vi "Digital_Counter_w_External_Clock_V2.vi"() -> ()   [LabVIEW 2020]
uses:
  <vilib>/Utility/error.llb/DialogType.ctl
  <vilib>/DAQmx/create/channels.llb/DAQmx Create Channel (CO-Pulse Generation-Frequency).vi
  <vilib>/DAQmx/configure/timing.llb/DAQmx Timing (Implicit).vi
panel:
  out "Feet Traveled":u64
  in  "stop":bool
  out "Pulse Count":u64
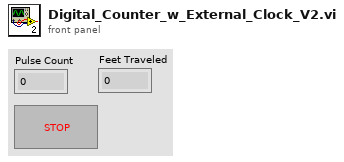
[diagram p1: front panel]
types:
  T1 = typedef "DialogType.ctl" = u16
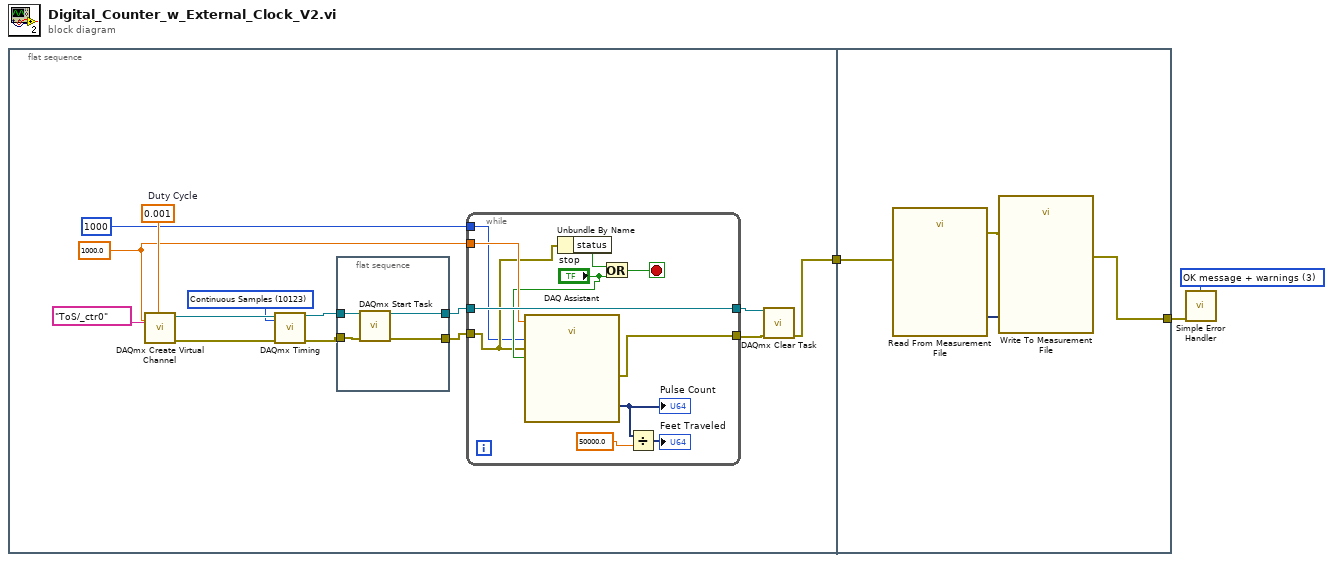
[diagram p0: block diagram]
diagram:
  w3 = T1 3 items=["no dialog", "OK message", "continue or stop message", "OK message + warnings", "continue/stop + warnings"] ("type of dialog (OK msg:1)")
  n1 = flat-sequence {
    tunnel: [w4] -> w2
    tunnel: w2 -> [w34]
    tunnel: [w33] -> w1
    frame #0 {
      w7 = 1000.0 ("Rate (Hz)")
      w13 = 0.001  # Duty Cycle
      w15 = 10123 items=["Finite Samples"=10178, "Continuous Samples"=10123] ("sample mode")
      n2 = call-poly <vilib>:"DAQmx Create Virtual Channel.vi"("frequency"=w7, "duty cycle"=w13, "counter"=tag "ToS/_ctr0" ("Sample Clock Src")) -> ("task out"=w16:refnum<k21>, "error out"=w17:errorcluster)  [unwired: 11 in]
      n3 = call-poly <vilib>:"DAQmx Timing.vi"("task/channels in"=w16, "sample mode"=w15, "error in"=w17) -> ("task out"=w12:refnum<k21>, "error out"=w11:errorcluster)  [unwired: 11 in]
      n4 = flat-sequence {
        tunnel: w12 -> [w32]
        tunnel: w11 -> [w31]
        tunnel: [w30] -> w10
        tunnel: [w29] -> w9
        frame #0 {
          n5 = call <vilib>:"DAQmx Start Task.vi"("task/channels in"=w32, "error in"=w31) -> ("task out"=w30:refnum<k21>, "error out"=w29:errorcluster)  [unwired: 12 in]
        }
      }
      n6 = while {
        tunnel: w10 -> [w28]
        tunnel: w9 -> [w24]
        tunnel: [w28] -> w8
        tunnel: w7 -> [w27]
        tunnel: 1000 ("number of samples") -> [w23]
        tunnel: [w21] -> w5
        stop <- w22 stop-if-true
        n7 = call "DAQ Assistant"("rate"=w27, "number of samples"=w23, "error in"=w24, "stop (F)"="stop") -> ("data"=w19:dynamicdata, "error out"=w21:errorcluster)  [unwired: 12 in, 2 out]
        "Pulse Count" <- w19
        n8 = Unbundle By Name(w24) -> ("status"=w26:bool)
        n9 = Or(x=w26, y="stop") -> (x .or. y?=w22:bool)
        n10 = Divide(x=w19, y=50000.0) -> (x/y=→"Feet Traveled":dynamicdata)
      }
      n11 = call <vilib>:"DAQmx Clear Task.vi"("task in"=w8, "error in"=w5) -> ("error out"=w4:errorcluster)  [unwired: 13 in]
    }
    frame #1 {
      n12 = call "Read From Measurement File"("error in (no error)"=w34) -> ("error out"=w35:errorcluster, "Signals"=w36:dynamicdata)  [unwired: 5 in, 4 out]
      n13 = call "Write To Measurement File"("Signals"=w36, "error in (no error)"=w35) -> ("error out"=w33:errorcluster)  [unwired: 15 in, 2 out]
    }
  }
  n14 = call <vilib>:"Simple Error Handler.vi"("type of dialog (OK msg:1)"=w3, "error in (no error)"=w1) -> ()  [unwired: 3 in, 5 out]
